vi "InitMain-UV-visSD.vi"() -> (0 "error out":errorcluster)   [LabVIEW 2015]
uses:
  atmcd32d.llb/HSSpeed_type typedef.ctl
  atmcd32d.llb/ReadMode_mode typedef.ctl
  atmcd32d.llb/TriggerMode_mode typedef.ctl
  AcquisitionMode_mode typedef.ctl
panel:
  in  "mode":T1=enum."External"
  in  "readout  mode":T2=enum."Multi-Track"
  in  "type":T3
  in  "directory (\"\")":string
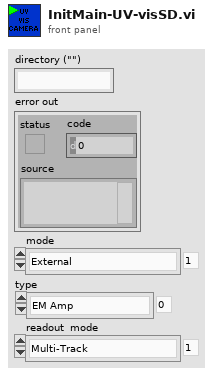
[diagram p1: front panel]
types:
  T1 = typedef "TriggerMode_mode typedef.ctl" = enum16{"Internal", "External", "N/A (2)", "N/A (3)", "N/A (4)", "N/A (5)", "External Start", "External Exposure (Bulb)", "N/A (8)", "External FVB EM", "Software", "N/A (11)", "External Charge Shifting"}
  T2 = typedef "ReadMode_mode typedef.ctl" = enum16{"Full Vertical Binning", "Multi-Track", "Random-Track", "Single-Track", "Image"}
  T3 = typedef "HSSpeed_type typedef.ctl" = enum16{"EM Amp", "Conventional Amp"}
  T4 = typedef "AcquisitionMode_mode typedef.ctl" = enum16{"Reserved (0)", "Single Scan", "Accumulate", "Kinetics", "Fast Kinetics", "Run Till Abort for non-Frame Transfer", "Frame Transfer", "Run Till Abort for Frame Transfer", "Reserved (8)", "Time Delayed Integration"}
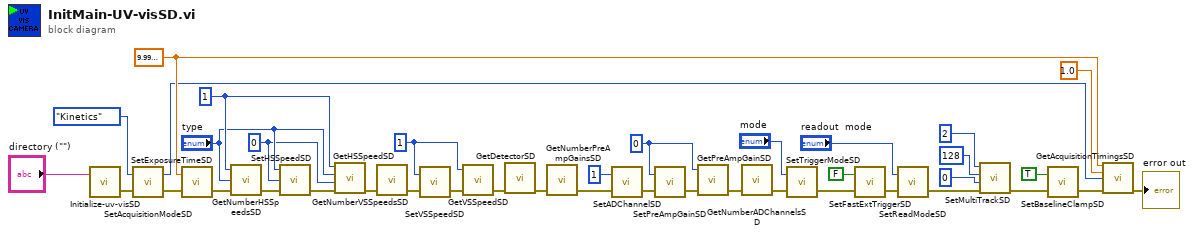
[diagram p0: block diagram]
diagram:
  w7 = 0 ("index HSSpeed")
  w29 = 1 ("index VSSpeed")
  w25 = 0 ("index preamp gain")
  w24 = sgl 0.0001 ("time")
  w32 = 1 ("channel HSSpeed")
  n1 = call "Initialize-uv-visSD.vi"("directory (\"\")"="directory (\"\")") -> ("error out"=w5:errorcluster)  [unwired: 1 in, 1 out]
  n2 = call "SetAcquisitionModeSD.vi"("error in (no error)"=w5, "mode"=AcquisitionMode_mode_typedef."Kinetics") -> ("error out"=w10:errorcluster, "DLL error code"=w11:u32)
  n3 = call "SetExposureTimeSD.vi"("error in (no error)"=w10, "time"=w24) -> ("error out"=w22:errorcluster)  [unwired: 1 out]
  n4 = call "GetNumberHSSpeedsSD.vi"("error in (no error)"=w22, "type"="type", "channel"=w32) -> ("error out"=w33:errorcluster)  [unwired: 2 out]
  n5 = call "SetHSSpeedSD.vi"("error in (no error)"=w33, "index"=w7, "type"="type") -> ("error out"=w34:errorcluster)  [unwired: 1 in, 1 out]
  n6 = call "GetHSSpeedSD.vi"("error in (no error)"=w34, "index"=w7, "type"="type", "channel"=w32) -> ("error out"=w21:errorcluster)  [unwired: 1 in, 2 out]
  n7 = call "GetNumberVSSpeedsSD.vi"("error in (no error)"=w21) -> ("error out"=w31:errorcluster)  [unwired: 2 in, 2 out]
  n8 = call "SetVSSpeedSD.vi"("error in (no error)"=w31, "index"=w29) -> ("error out"=w30:errorcluster)  [unwired: 1 out]
  n9 = call "GetVSSpeedSD.vi"("error in (no error)"=w30, "index"=w29) -> ("error out"=w20:errorcluster)  [unwired: 1 in, 2 out]
  n10 = call "GetDetectorSD.vi"("error in (no error)"=w20) -> ("error out"=w19:errorcluster)  [unwired: 3 in, 3 out]
  n11 = call "GetNumberPreAmpGainsSD.vi"("error in (no error)"=w19) -> ("error out"=w9:errorcluster)  [unwired: 2 in, 2 out]
  n12 = call "SetADChannelSD.vi"("error in (no error)"=w9, "channel"=1) -> ("error out"=w8:errorcluster)  [unwired: 1 out]
  n13 = call "SetPreAmpGainSD.vi"("error in (no error)"=w8, "index"=w25) -> ("error out"=w36:errorcluster)  [unwired: 1 out]
  n14 = call "GetPreAmpGainSD.vi"("error in (no error)"=w36, "index"=w25) -> ("error out"=w14:errorcluster)  [unwired: 1 in, 2 out]
  n15 = call "GetNumberADChannelsSD.vi"("error in (no error)"=w14) -> ("error out"=w18:errorcluster)  [unwired: 2 in, 2 out]
  n16 = call "SetTriggerModeSD.vi"("error in (no error)"=w18, "mode"="mode") -> ("error out"=w39:errorcluster)  [unwired: 1 out]
  n17 = call "SetFastExtTriggerSD.vi"("error in (no error)"=w39, "mode"=FALSE ("Fast external mode")) -> ("error out"=w17:errorcluster)  [unwired: 1 out]
  n18 = call "SetReadModeSD.vi"("error in (no error)"=w17, "mode"="readout  mode") -> ("error out"=w35:errorcluster)  [unwired: 1 out]
  n19 = call "SetMultiTrackSD.vi"("error in (no error)"=w35, "offset"=0, "height"=128, "number"=2) -> ("error out"=w3:errorcluster)  [unwired: 3 out]
  n20 = call "SetBaselineClampSD.vi"("error in (no error)"=w3, "state"=TRUE ("Base line Clamp")) -> ("error out"=w2:errorcluster)  [unwired: 1 out]
  n21 = call "GetAcquisitionTimingsSD.vi"("exposure input"=w24, "accumulate input"=sgl 1.0, "kinetic input"=w11, "error in (no error)"=w2) -> ("error out"=→"error out":errorcluster)  [unwired: 7 in, 4 out]
